vi "Get Templates Directory Path.vi"() -> (3 "Templates Directory":path)   [LabVIEW 2018, in "Create New Assert Tester.lvclass"]
uses:
  Create New Assert Tester.lvclass
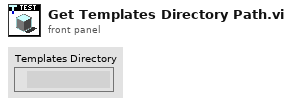
[diagram p1: front panel]
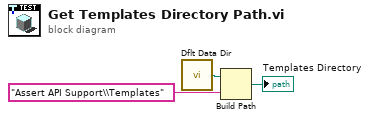
[diagram p0: block diagram]
diagram:
  n1 = call <vilib>:"Dflt Data Dir.vi"() -> ("App:Default Data Directory"=w3:path)
  n2 = Build Path(base path=w3, name or relative path="Assert API Support\\Templates") -> (appended path=→"Templates Directory":path)
